vi "Save File DOE Create Filename.vi"(8 "error in (no error)":errorcluster, 9 "Lab ID":string, 10 "TR Number":string, 11 "Save File Path":path) -> (0 "error out":errorcluster, 1 "Debug File Path":path, 2 "Data File Path":path, 3 "Save Folder Path":path)   [LabVIEW 2016]
panel:
  out "Debug File Name":string
  out "Data File Name":string
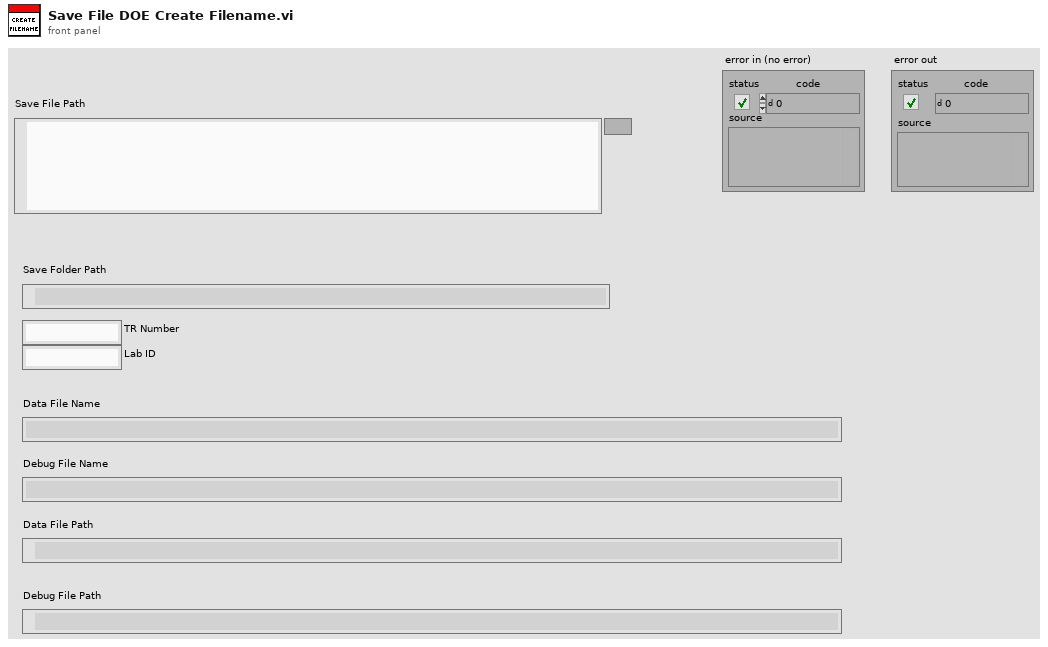
[diagram p1: front panel]
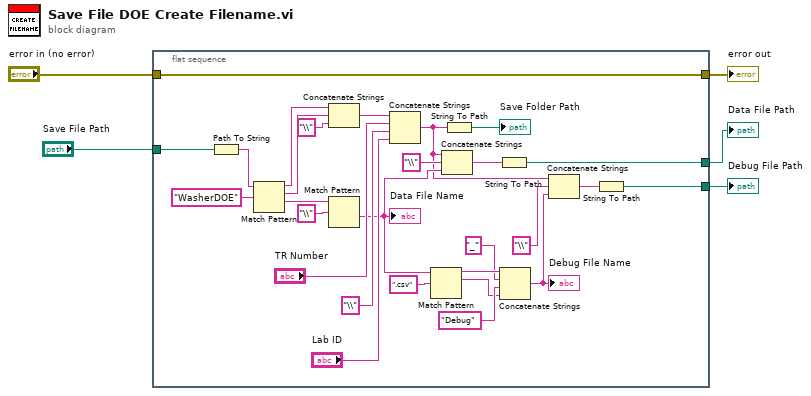
[diagram p0: block diagram]
diagram:
  n1 = flat-sequence {
    tunnel: "Save File Path" -> [w33]
    tunnel: "error in (no error)" -> [w8]
    tunnel: [w8] -> w3
    tunnel: [w7] -> w2
    tunnel: [w6] -> w1
    frame #0 {
      n2 = Path To String(path=w33) -> (string=w32:string)
      n3 = Match Pattern(string=w32, regular expression="WasherDOE") -> (before substring=w29:string, match substring=w30:string, after substring=w22:string)  [unwired: 1 in, 1 out]
      n4 = Concatenate Strings(w29, w30, "\\" ("string")) -> (w27:string)
      n5 = Match Pattern(string=w22, regular expression="\\" ("string")) -> (after substring=w14:string)  [unwired: 1 in, 3 out]
      "Data File Name" <- w14
      n6 = Concatenate Strings(w27, "TR Number", "\\" ("string"), "Lab ID") -> (w13:string)
      n7 = Match Pattern(string=w14, regular expression=".csv") -> (before substring=w19:string, match substring=w16:string)  [unwired: 1 in, 2 out]
      n8 = Concatenate Strings(w13, "\\" ("string"), w14) -> (w10:string)
      n9 = String To Path(string=w13) -> (path=→"Save Folder Path":path)
      n10 = String To Path(string=w10) -> (path=w7:path)
      n11 = Concatenate Strings(w19, "_" ("string"), "Debug" ("string"), w16) -> (w11:string)
      "Debug File Name" <- w11
      n12 = Concatenate Strings(w13, "\\" ("string"), w11) -> (w9:string)
      n13 = String To Path(string=w9) -> (path=w6:path)
    }
  }
  "error out" <- w3
  "Data File Path" <- w2
  "Debug File Path" <- w1
